vi "Count Character.vi"(6 "Amount":i64, 7 "Character":string, 11 "Count In":i64[](array[numeric])) -> (3 "Count Out":i64[](array[numeric]))   [LabVIEW 2021]
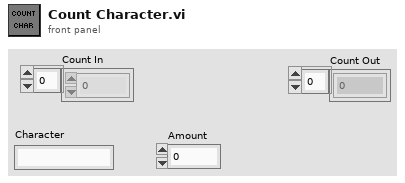
[diagram p1: front panel]
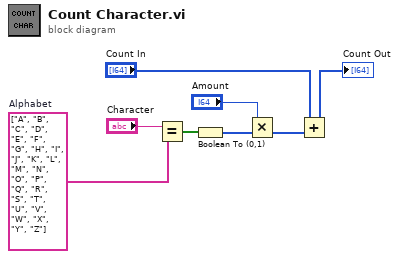
[diagram p0: block diagram]
diagram:
  w3 = string[] ["A", "B", "C", "D", "E", "F", "G", "H", "I", "J", "K", "L", "M", "N", "O", "P", "Q", "R", "S", "T", "U", "V", "W", "X", "Y", "Z"]  # Alphabet
  n1 = Equal?(x="Character", y=w3) -> (x = y?=w7:bool[])
  n2 = Boolean To (0,1)(Boolean=w7) -> (0, 1=w6:i16[])
  n3 = Multiply(x="Amount", y=w6) -> (x*y=w2:i64[])
  n4 = Add(x="Count In", y=w2) -> (x+y=→"Count Out":i64[])
